vi "User Process Test.vi"() -> ()   [LabVIEW 2017, in "Tank Controller Logic tests.lvlib"]
uses:
  Tank Controller Logic tests.lvlib
  module/execution/parameter user data.ctl
  module/execution/result user data.ctl
  module/execution/Tank Controller Logic runtime.lvclass
panel:
  in  "stop":bool
  out "Results from processing":T1
  out "error out":errorcluster
  in  "Parameters to process":T2
  in  "error in":errorcluster
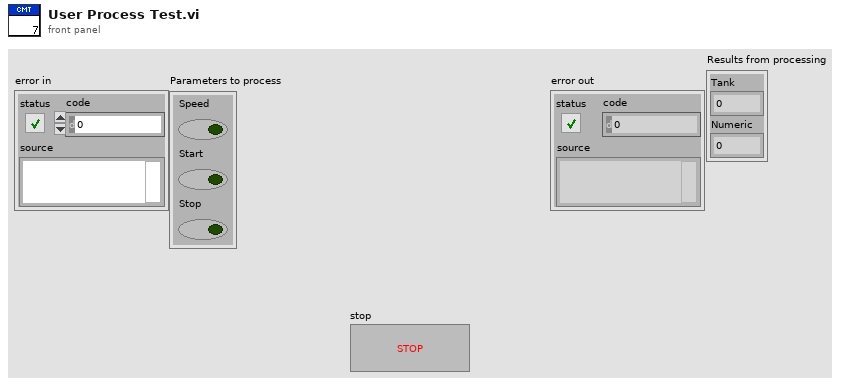
[diagram p1: front panel]
types:
  T1 = typedef "Tank Controller Logic runtime.lvclass/result user data.ctl" = cluster{"Tank":dbl, "Numeric":dbl}
  T2 = typedef "Tank Controller Logic runtime.lvclass/parameter user data.ctl" = cluster{"Speed":bool, "Start":bool, "Stop":bool}
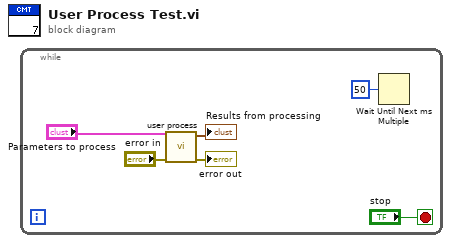
[diagram p0: block diagram]
diagram:
  n1 = while {
    stop <- "stop" stop-if-true
    n2 = call "user process.vi"("error in"="error in", "Parameters to process"="Parameters to process") -> ("error out"=→"error out":errorcluster, "Results from processing"=→"Results from processing":T1)  [unwired: 8 in]
    n3 = Wait Until Next ms Multiple(millisecond multiple=u32 50) -> ()  [unwired: 1 out]
  }
